vi "get date time string for filename.vi"() -> (3 "time string":string)   [LabVIEW 2020]
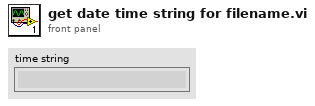
[diagram p1: front panel]
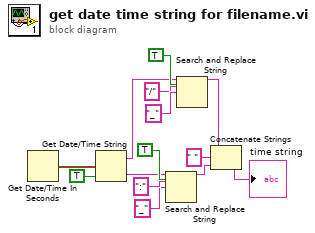
[diagram p0: block diagram]
diagram:
  n1 = Get Date/Time In Seconds() -> (seconds since 1Jan1904=w14:timestamp)
  n2 = Get Date/Time String(seconds (now)=w14, want seconds? (F)=TRUE) -> (date string=w2:string, time string=w11:string)  [unwired: 1 in]
  n3 = Search and Replace String(replace all?=TRUE ("replace all? (F)"), input string=w11, search string=":", replace string="_" ("replace string (\"\")")) -> (result string=w7:string)  [unwired: 4 in, 3 out]
  n4 = Search and Replace String(replace all?=TRUE ("replace all? (F)"), input string=w2, search string="/", replace string="_" ("replace string (\"\")")) -> (result string=w1:string)  [unwired: 4 in, 3 out]
  n5 = Concatenate Strings(w1, " " ("string"), w7) -> (→"time string":string)
